vi "EFW_test.vi"() -> ()   [LabVIEW 2012]
uses:
  <userlib>/EFW_filter/EFW_filter.lvlib
panel:
  in  "unidirect":bool
  in  "calibrate":bool
  in  "wheel index":i32
  in  "target position":i8(knob) scale=0.0..10.0
  out "current position":i32
  in  "stop":bool
  in  "move":bool
  out "ID":i32
  out "connected wheel num":i32
  out "slot num":i32
  in  "错误输入（无错误）":errorcluster
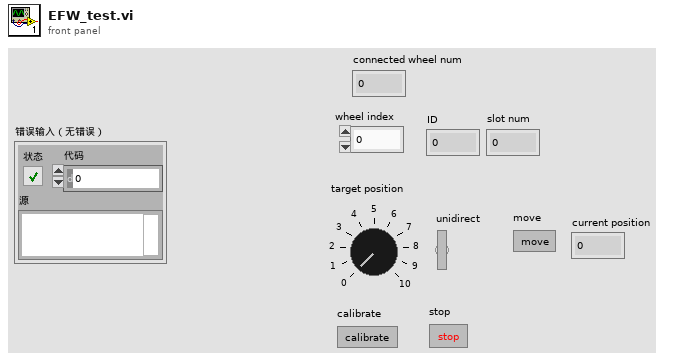
[diagram p1: front panel]
types:
  T1 = cluster{"ID":i32, "Name[0]":i8, "Name[1]":i8, "Name[2]":i8, "Name[3]":i8, "Name[4]":i8, "Name[5]":i8, "Name[6]":i8, "Name[7]":i8, "Name[8]":i8, "Name[9]":i8, "Name[10]":i8, "Name[11]":i8, "Name[12]":i8, "Name[13]":i8, "Name[14]":i8, "Name[15]":i8, "Name[16]":i8, "Name[17]":i8, "Name[18]":i8, "Name[19]":i8, "Name[20]":i8, "Name[21]":i8, "Name[22]":i8, "Name[23]":i8, "Name[24]":i8, "Name[25]":i8, "Name[26]":i8, "Name[27]":i8, "Name[28]":i8, "Name[29]":i8, "Name[30]":i8, "Name[31]":i8, "Name[32]":i8, "Name[33]":i8, "Name[34]":i8, "Name[35]":i8, "Name[36]":i8, "Name[37]":i8, "Name[38]":i8, "Name[39]":i8, "Name[40]":i8, "Name[41]":i8, "Name[42]":i8, "Name[43]":i8, "Name[44]":i8, "Name[45]":i8, "Name[46]":i8, "Name[47]":i8, "Name[48]":i8, "Name[49]":i8, "Name[50]":i8, "Name[51]":i8, "Name[52]":i8, "Name[53]":i8, "Name[54]":i8, "Name[55]":i8, "Name[56]":i8, "Name[57]":i8, "Name[58]":i8, "Name[59]":i8, "Name[60]":i8, "Name[61]":i8, "Name[62]":i8, "Name[63]":i8, "slotNum":i32}
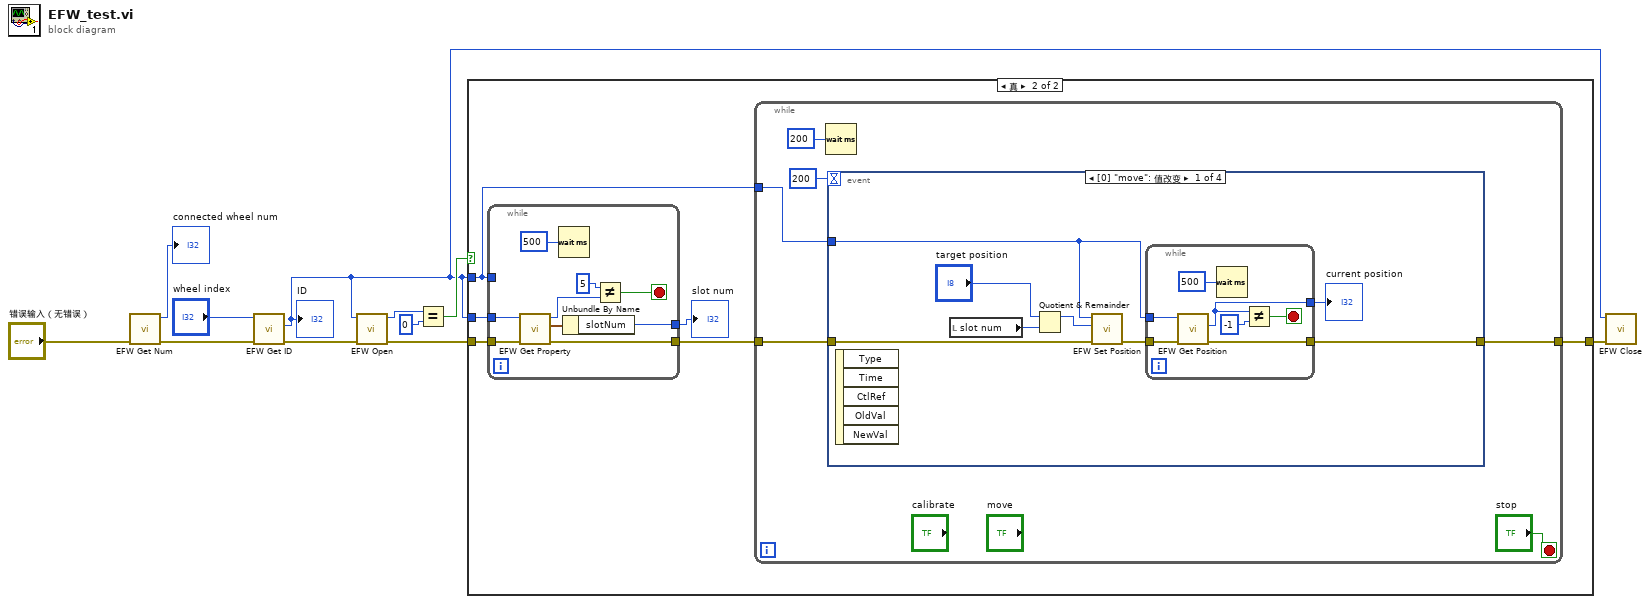
[diagram p0: block diagram]
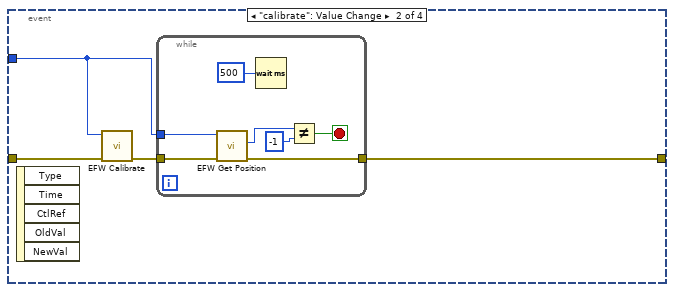
[diagram p3: hidden frame]
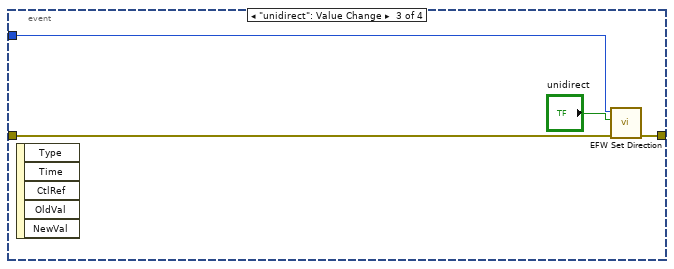
[diagram p4: hidden frame]
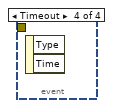
[diagram p5: hidden frame]
diagram:
  n1 = call <userlib>:"EFW Get Num.vi"("error in (no error)"="错误输入（无错误）") -> ("error out"=w7:errorcluster, "function return"=→"connected wheel num":i32)  [unwired: 9 in]
  n2 = call <userlib>:"EFW Get ID.vi"("error in (no error)"=w7, "index"="wheel index") -> ("error out"=w5:errorcluster, "ID out"=w1:i32)  [unwired: 7 in, 1 out]
  "ID" <- w1
  n3 = call <userlib>:"EFW Open.vi"("error in (no error)"=w5, "ID"=w1) -> ("error out"=w4:errorcluster, "function return"=w3:u32)  [unwired: 8 in]
  n4 = Equal?(x=w3, y=0) -> (x = y?=w10:bool)
  n5 = case shown="真" w10 {
    tunnel: w4 -> [w12 w18]
    tunnel: w1 -> [_ w15]
    tunnel: [w12 w14] -> w2
    tunnel: w1 -> [_ w13]
    frame False {
    }
    frame True {
      n6 = while {
        tunnel: w15 -> [_]
        tunnel: w18 -> [w60]
        tunnel: [w56] -> w16
        tunnel: [w59] -> w17
        tunnel: w13 -> [w58]
        stop <- w61 stop-if-true
        n7 = call <userlib>:"EFW Get Property.vi"("error in (no error)"=w60, "ID"=w58) -> ("error out"=w59:errorcluster, "pInfo out"=w57:T1, "function return"=w55:u32)  [unwired: 7 in]
        n8 = Wait (ms)(milliseconds to wait=500) -> ()  [unwired: 1 out]
        n9 = Unbundle By Name(w57) -> ("slotNum"=w56:i32)
        n10 = Not Equal?(x=5, y=w55) -> (x != y?=w61:bool)
      }
      "slot num" <- w16
      n11 = while {
        tunnel: w15 -> [w21]
        tunnel: w17 -> [w20]
        tunnel: [w22] -> w14
        stop <- "stop" stop-if-true
        n12 = Wait (ms)(milliseconds to wait=200) -> ()  [unwired: 1 out]
        n13 = event shown="[0] \"move\": 值改变" {
          selector: _ -> [_ _ _ _]
          dyn-events: _ -> [_ _ _ _]
          timeout: 200 -> [_ _ _ _]
          tunnel: w21 -> [w26 w42 w53 _]
          tunnel: w20 -> [w29 w40 w52 _]
          tunnel: [w30 w41 w51 _] -> w22
          event "move": Value Change {
            n14 = event-data() -> ()  [unwired: 1 in, 5 out]
            n15 = local read "slot num"() -> (w25:i32)
            n16 = Quotient & Remainder(x="target position", y=w25) -> (x-y*floor(x/y)=w27:i32)  [unwired: 1 out]
            n17 = call <userlib>:"EFW Set Position.vi"("error in (no error)"=w29, "Position"=w27, "ID"=w26) -> ("error out"=w28:errorcluster)  [unwired: 7 in, 1 out]
            n18 = while {
              tunnel: w28 -> [w36]
              tunnel: w26 -> [w33]
              tunnel: [w34] -> w31
              tunnel: [w35] -> w30
              stop <- w37 stop-if-true
              n19 = call <userlib>:"EFW Get Position.vi"("error in (no error)"=w36, "ID"=w33) -> ("error out"=w35:errorcluster, "pPosition out"=w34:i32)  [unwired: 7 in, 1 out]
              n20 = Wait (ms)(milliseconds to wait=500) -> ()  [unwired: 1 out]
              n21 = Not Equal?(x=w34, y=-1) -> (x != y?=w37:bool)
            }
            "current position" <- w31
          }
          event "calibrate": Value Change {
            n22 = event-data() -> ()  [unwired: 1 in, 5 out]
            n23 = call <userlib>:"EFW Calibrate.vi"("error in (no error)"=w40, "ID"=w42) -> ("error out"=w43:errorcluster)  [unwired: 8 in, 1 out]
            n24 = while {
              tunnel: w43 -> [w47]
              tunnel: w42 -> [w44]
              tunnel: [w46] -> w41
              stop <- w48 stop-if-true
              n25 = call <userlib>:"EFW Get Position.vi"("error in (no error)"=w47, "ID"=w44) -> ("error out"=w46:errorcluster, "pPosition out"=w45:i32)  [unwired: 7 in, 1 out]
              n26 = Wait (ms)(milliseconds to wait=500) -> ()  [unwired: 1 out]
              n27 = Not Equal?(x=w45, y=-1) -> (x != y?=w48:bool)
            }
          }
          event "unidirect": Value Change {
            n28 = event-data() -> ()  [unwired: 1 in, 5 out]
            n29 = call <userlib>:"EFW Set Direction.vi"("error in (no error)"=w52, "bUnidirectional"="unidirect", "ID"=w53) -> ("error out"=w51:errorcluster)  [unwired: 7 in, 1 out]
          }
          event Timeout {
            n30 = event-data() -> ()  [unwired: 1 in, 2 out]
          }
        }
      }
    }
  }
  n31 = call <userlib>:"EFW Close.vi"("error in (no error)"=w2, "ID"=w1) -> ()  [unwired: 8 in, 2 out]
